vi "mono_connect.vi"(3 "error in":errorcluster, 4 "monoDrive Control Port":i32, 5 "monoDrive Simulator IP":string) -> (0 "error out":errorcluster, 2 "monoDrive Connection":refnum<k5>)   [LabVIEW 2018, in "monoDrive.lvlib"]
uses:
  monoDrive.lvlib
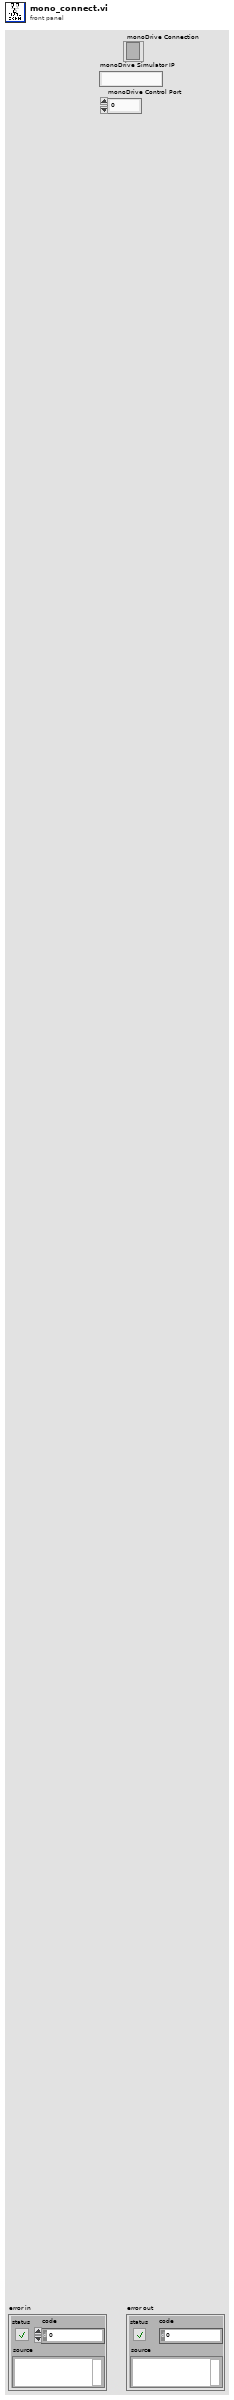
[diagram p1: front panel]
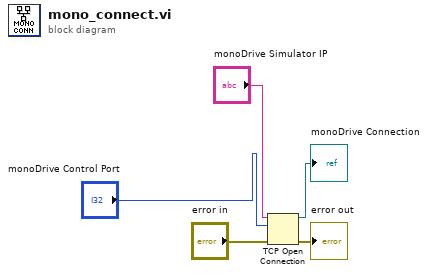
[diagram p0: block diagram]
diagram:
  n1 = TCP Open Connection(address="monoDrive Simulator IP", remote port or service name="monoDrive Control Port", error in (no error)="error in") -> (connection ID=→"monoDrive Connection":refnum<k5>, error out=→"error out":errorcluster)  [unwired: 2 in]
